vi "acquireValue.vi"(8 "error in (no error)":errorcluster, 10 "nextSample?":bool, 11 "position in":refnum<class "position.lvclass">) -> (0 "error out":errorcluster, 1 "function return":i32, 2 "variantData":variant, 3 "position out":refnum<class "position.lvclass">)   [LabVIEW 2016, in "SALLV_AtDome_Messaging.lvlib" / "position.lvclass"]
uses:
  position.lvclass
  ts_sallv_AtDome/SALLV_AtDome.lvlib
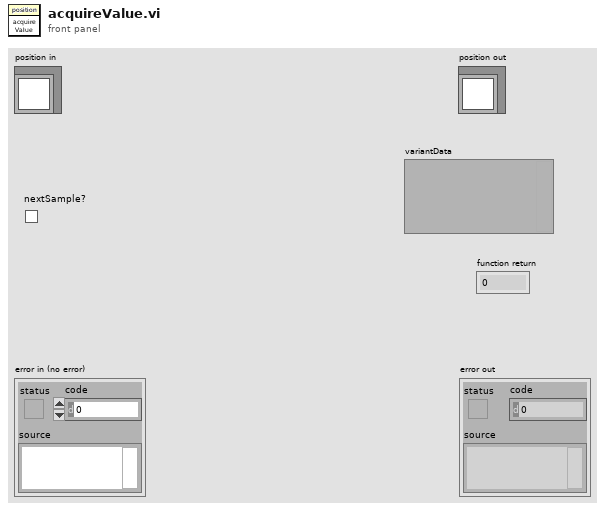
[diagram p1: front panel]
types:
  T1 = typedef "SALLV_AtDome.lvlib/position.ctl" = cluster{"dropoutOpeningPercentage":sgl, "mainDoorOpeningPercentage":sgl, "azimuthPosition":dbl, "dropoutOpeningPercentageSet":sgl, "mainDoorOpeningPercentageSet":sgl, "azimuthPositionSet":dbl}
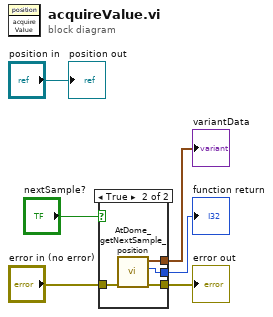
[diagram p0: block diagram]
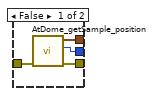
[diagram p2: hidden frame]
diagram:
  n1 = case shown="True" "nextSample?" {
    tunnel: "error in (no error)" -> [w10 w14]
    tunnel: [w9 w13] -> w2
    tunnel: [w7 w11] -> w3
    tunnel: [w8 w12] -> w4
    frame False {
      n2 = call "AtDome_getSample_position.vi"("error in (no error)"=w10) -> ("error out"=w9:errorcluster, "function return"=w8:i32, "position_Ctl out"=w7:T1)  [unwired: 8 in]
    }
    frame True {
      n3 = call "AtDome_getNextSample_position.vi"("error in (no error)"=w14) -> ("error out"=w13:errorcluster, "function return"=w12:i32, "position_Ctl out"=w11:T1)  [unwired: 8 in]
    }
  }
  "error out" <- w2
  "variantData" <- w3
  "function return" <- w4
  "position out" <- "position in"
